vi "Install Package.vi"(8 "error in":errorcluster, 10 "version":string, 11 "package name":string) -> (0 "error out":errorcluster, 3 "package name out":string)   [LabVIEW 2014, in "NIPM_API.lvlib"]
doc: "Installs the specified package on this computer.\n\nversion input:\nIf the version input is left unwired and no version of the package is currently installed, this VI will install the latest version of the package available from the registered feeds on the computer.\nIf the version input is left unwired and any version of the package is currently installed, this VI will output an error.\n\nIf the version input is wired and a different version of the package is installed, this VI will upgrade or downgrade the package to the specified version.\nIf the version input is wired and the specified version of the package is already installed, this VI will output an error.\n\nNOTE: This VI does not work when the package installation requires admin priviledges (e.g. package installs files to Program Files directory)."
uses:
  NIPM_API.lvlib
panel:
  out "command line standard output":string
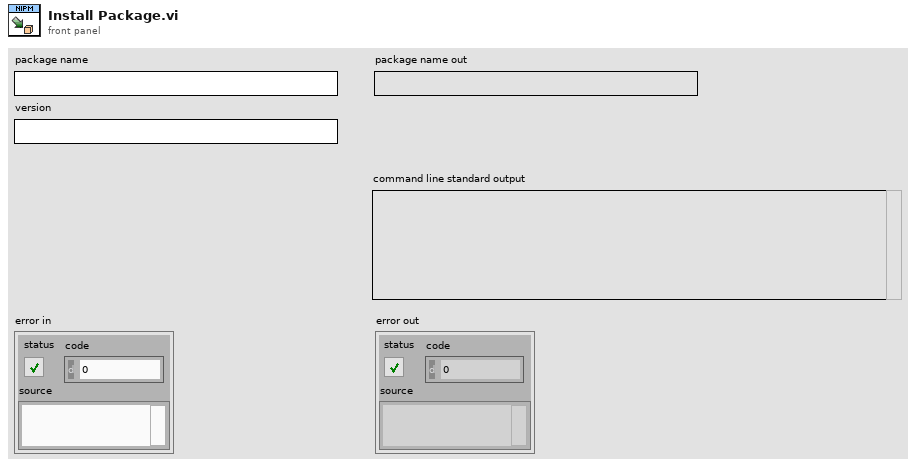
[diagram p1: front panel]
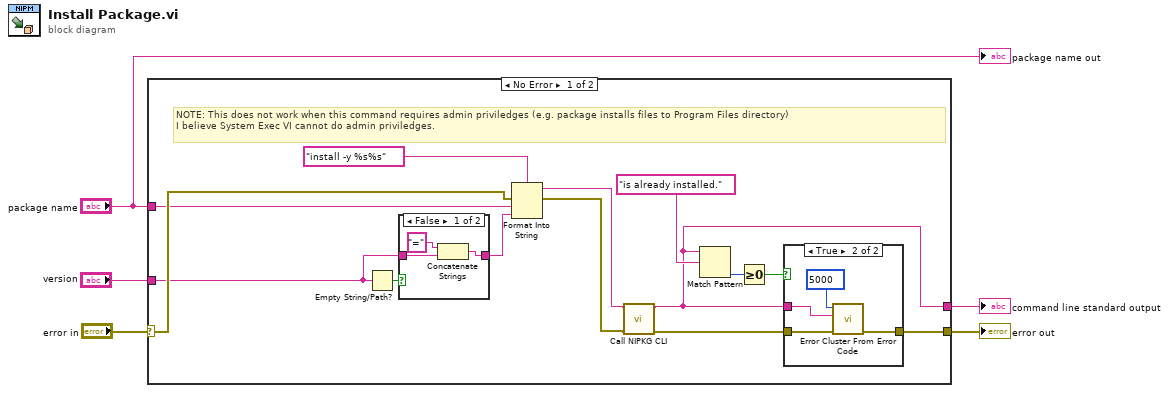
[diagram p0: block diagram]
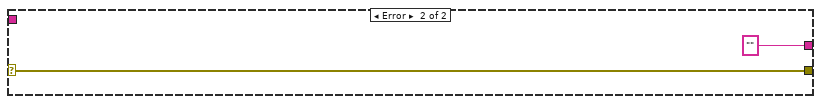
[diagram p4: hidden frame]
diagram:
  n1 = case shown="No Error" "error in" {
    selector: "error in" -> [w18 w30]
    tunnel: [w8 "" ("standard output")] -> w4
    tunnel: [w9 w30] -> w3
    tunnel: "package name" -> [w7 _]
    tunnel: "version" -> [w6 _]
    frame No Error {
      # "NOTE: This does not work when this command requires admin priviledges (e.g. package installs files to Program Files directory)\nI believe System Exec VI cannot do admin priviledges."
      n2 = Empty String/Path?(string/path=w6) -> (empty?=w17:bool)
      n3 = case shown="False" w17 {
        tunnel: w6 -> [w27 w28]
        tunnel: [w25 w28] -> w16
        frame False {
          n4 = Concatenate Strings("=" ("string"), w27) -> (w25:string)
        }
        frame True {
        }
      }
      n5 = Format Into String(format string="install -y %s%s", error in=w18, w7, w16) -> (resulting string=w14:string, error out=w15:errorcluster)  [unwired: 1 in]
      n6 = call "Call NIPKG CLI.vi"("error in (no error)"=w15, "command"=w14) -> ("error out"=w10:errorcluster, "command line standard output"=w8:string)  [unwired: 8 in]
      n7 = Match Pattern(string=w8, regular expression="is already installed.") -> (offset past match=w12:i32)  [unwired: 1 in, 3 out]
      n8 = Greater Or Equal To 0?(x=w12) -> (x >= 0?=w11:bool)
      n9 = case shown="True" w11 {
        tunnel: w10 -> [w20 w23]
        tunnel: [w20 w22] -> w9
        tunnel: w8 -> [_ w21]
        frame False {
        }
        frame True {
          n10 = call <vilib>:"Error Cluster From Error Code.vi"("error in (no error)"=w23, "error message (\"\")"=w21, "error code (0)"=5000) -> ("error out"=w22:errorcluster)  [unwired: 6 in]
        }
      }
    }
    frame Error {
    }
  }
  "error out" <- w3
  "command line standard output" <- w4
  "package name out" <- "package name"
